vi "RT Temperature Thold File Path.vi"() -> (3 "Cfg File Path out":path)   [LabVIEW 2015, in "Tool Cfg.lvlib"]
uses:
  Tool Cfg.lvlib
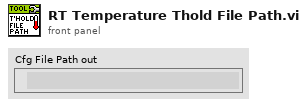
[diagram p1: front panel]
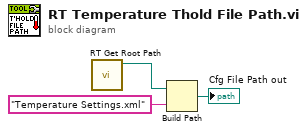
[diagram p0: block diagram]
diagram:
  n1 = call "RT Get Root Path.vi"() -> ("Root Path out"=w1:path)  [unwired: 11 in]
  n2 = Build Path(base path=w1, name or relative path="Temperature Settings.xml" ("Tool Cfg Cluster XML Filename")) -> (appended path=→"Cfg File Path out":path)
